vi "Configuration 1.0 Finalize.vi"(8 "error in (no error)":errorcluster, 10 "dsf version (1.0)":T2={"major"=1, "minor"=0, "fix"=0, "build"=""}, 11 "framework configuration 1.0":T1) -> (0 "error out":errorcluster, 2 "final dsf version":T2, 3 "dsf configuration json":string)   [LabVIEW 2017, in "DSF Core.lvlib" / "Configuration Session.lvclass"]
uses:
  Configuration Session.lvclass
  Typedefs/DSF Version Info.ctl
  DSF Core.lvlib
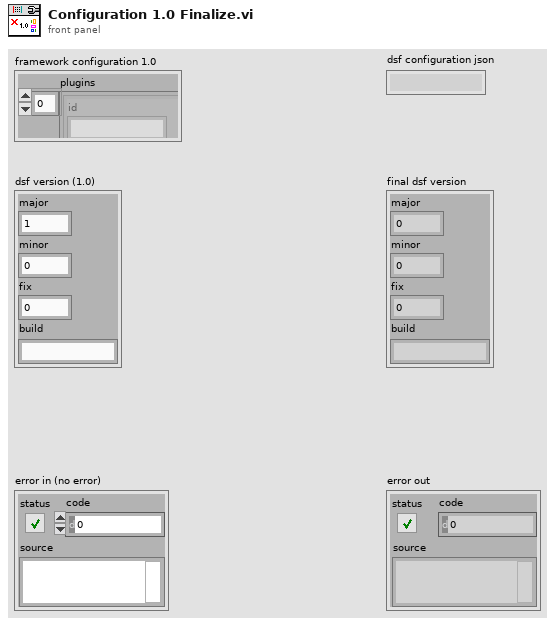
[diagram p1: front panel]
types:
  T1 = cluster{"plugins":cluster{"id":string, "values":cluster{"components":string[], "timing":cluster{"priority":u64, "decimation":u64, "offset":u64}, "group ids":string[], "settings id":string, "threads":cluster{"buffer converter settings":cluster{"key":string, "value":string}[], "transceiver settings":cluster{"key":string, "value":string}[], "custom settings":cluster{"key":string, "value":string}[], "processor":i32, "priority offset":i16}[]}}[], "groups":cluster{"id":string, "values":cluster{"direction":i32, "timing":cluster{"priority":u64, "decimation":u64, "offset":u64}, "transfer ids":string[], "settings id":string, "thread":i32, "timeout behavior":u8}}[], "transfers":cluster{"id":string, "values":cluster{"byte order":i32, "channel ids":string[], "settings id":string}}[], "channels":cluster{"id":string, "values":cluster{"string buffer offset":u64, "string data type":i32, "engine data type":i32, "settings id":string, "units":string}}[], "settings":cluster{"id":string, "values":cluster{"key":string, "value":string}[]}[]}
  T2 = typedef "DSF Core.lvlib/DSF Version Info.ctl" = cluster{"major":u32, "minor":u32, "fix":u32, "build":string}
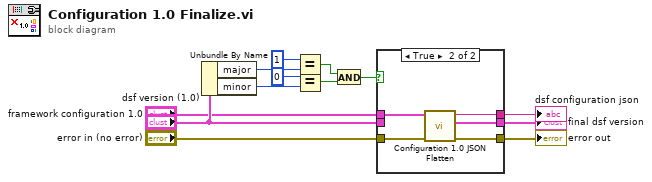
[diagram p0: block diagram]
diagram:
  n1 = Unbundle By Name("dsf version (1.0)") -> ("major"=w12:u32, "minor"=w13:u32)
  n2 = Equal?(x=u32 1, y=w12) -> (x = y?=w8:bool)
  n3 = Equal?(x=u32 0, y=w13) -> (x = y?=w9:bool)
  n4 = And(x=w8, y=w9) -> (x .and. y?=w7:bool)
  n5 = case shown="True" w7 {
    tunnel: "error in (no error)" -> [w14 w18]
    tunnel: "framework configuration 1.0" -> [_ w19]
    tunnel: [w14 w17] -> w5
    tunnel: "dsf version (1.0)" -> [_ _]
    tunnel: [_ w15] -> w4
    tunnel: [_ w16] -> w2
    frame False {
      # "Unknown version."
    }
    frame True {
      n6 = call "Configuration 1.0 JSON Flatten.vi"("error in (no error)"=w18, "framework configuration 1.0"=w19) -> ("error out"=w17:errorcluster, "dsf version"=w16:T2, "dsf configuration json"=w15:string)  [unwired: 7 in]
    }
  }
  "dsf configuration json" <- w4
  "error out" <- w5
  "final dsf version" <- w2
